vi "Open.vi"(8 "error in (no error)":errorcluster, 10 "PhyAxis":u16, 11 "DeviceNumber":u32=1644167168 format="0x%x") -> (0 "error out":errorcluster)   [LabVIEW 2020, in "输出轴伺服.lvlib"]
uses:
  Servo_global.vi
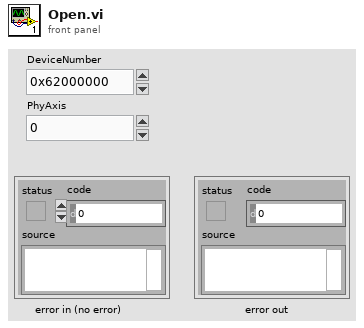
[diagram p1: front panel]
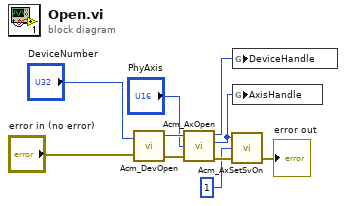
[diagram p0: block diagram]
diagram:
  n1 = call <userlib>:"Acm_DevOpen.vi"("error in (no error)"="error in (no error)", "DeviceNumber"="DeviceNumber") -> ("error out"=w6:errorcluster, "DeviceHandle"=w9:u32)  [unwired: 1 out]
  n2 = call <userlib>:"Acm_AxOpen.vi"("error in (no error)"=w6, "PhyAxis"="PhyAxis", "DeviceHandle"=w9) -> ("error out"=w4:errorcluster, "AxisHandle"=w1:u32, "DeviceHandle"=w5:u32)  [unwired: 1 out]
  n3 = call <userlib>:"Acm_AxSetSvOn.vi"("error in (no error)"=w4, "OnOff"=u32 1, "AxisHandle"=w1) -> ("error out"=→"error out":errorcluster)  [unwired: 2 out]
  n4 = global write "Servo_global.vi" "DeviceHandle"(w5) -> ()
  n5 = global write "Servo_global.vi" "AxisHandle"(w1) -> ()
